vi "niSYS - SA - UTIL - IQ Waveform to TDMS.vi"(8 "error in (no error)":errorcluster, 9 "File Path or Name":path, 11 "Complex Waveform":cluster{"x0":dbl, "dx":dbl, "y":cdb[]} {"y" format="%.2f"; "dx" format="%^.2e"; "x0" format="%^.2e"}) -> (0 "error out":errorcluster)   [LabVIEW 2020]
doc: "(c) Copyright 2006, National Instruments, Inc. This VI may not be duplicated, sold, or distributed without written consent from National Instruments."
panel:
  in  "Waveform Name":string="test"
  in  "Headroom, dB (-1 = Auto)":dbl format="%.1f"
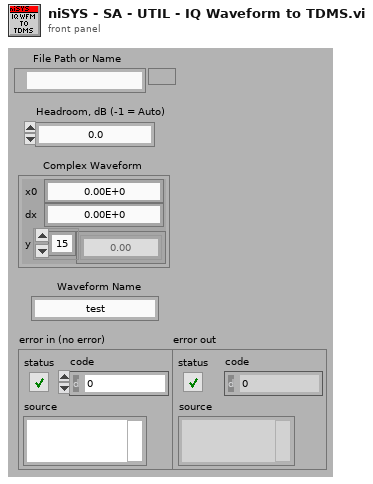
[diagram p1: front panel]
types:
  T1 = enum16{"open", "open or create", "create or replace", "create", "open (read-only)"}
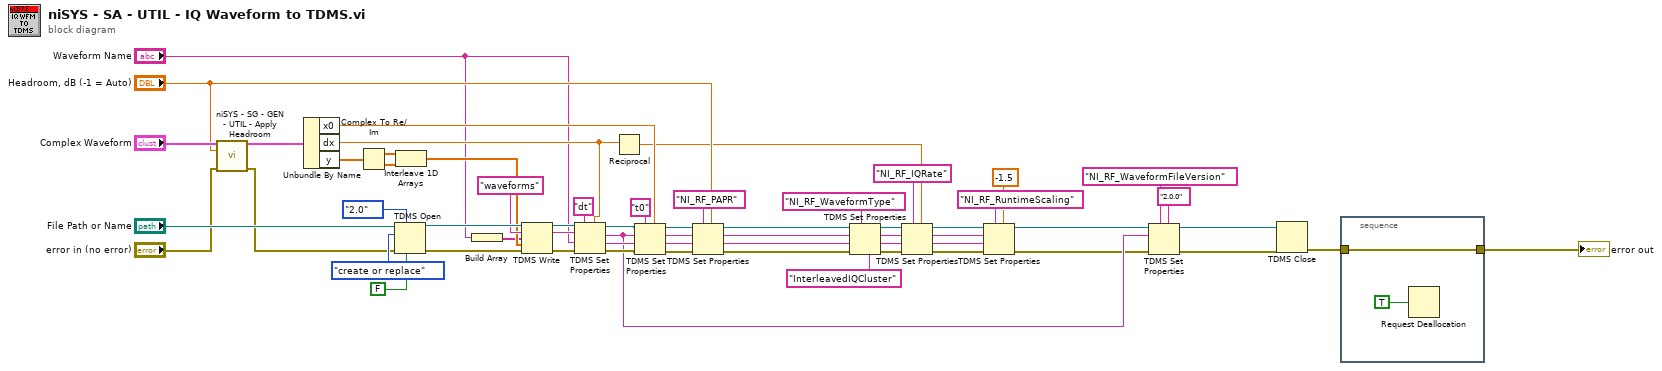
[diagram p0: block diagram]
diagram:
  n1 = call "niSYS - SG - GEN - UTIL - Apply Headroom.vi"("Complex Signal In"="Complex Waveform", "Headroom, dB (-1 = Auto)"="Headroom, dB (-1 = Auto)", "error in (no error)"="error in (no error)") -> ("Complex Signal Out"=w32:cluster{"x0":dbl, "dx":dbl, "y":cdb[]}, "error out"=w29:errorcluster)  [unwired: 10 in, 1 out]
  n2 = Unbundle By Name(w32) -> ("x0"=w36:dbl, "dx"=w27:dbl, "y"=w37:cdb[])
  n3 = Complex To Re/Im(x + iy=w37) -> (x=w39:dbl[], y=w38:dbl[])
  n4 = TDMS Open(6:FALSE ("disable buffering? (T)"), 7:enum16{"1.0", "2.0"}."2.0" ("file format version (2.0)"), 8:w29, 10:T1."create or replace" ("operation (0:open)"), 11:"File Path or Name") -> (0:w51:errorcluster, 3:w52:refnum<k34>)  [unwired: 2 in]
  n5 = Interleave 1D Arrays(w39, w38) -> (w25:dbl[])
  n6 = Build Array("Waveform Name") -> (w19:string[])
  n7 = TDMS Write(0:w52, 5:"waveforms" ("group name"), 7:w19, 9:w25, 11:w51) -> (4:w53:refnum<k34>, 6:w54:string, 15:w28:errorcluster)  [unwired: 1 in, 1 out]
  n8 = TDMS Set Properties(5:w27, 7:"dt", 8:w28, 9:"Waveform Name", 10:w54, 11:w53) -> (0:w49:errorcluster, 1:w44:string, 2:w9:string, 3:w50:refnum<k34>)
  n9 = Reciprocal(x=w27) -> (1/x=w26:dbl)
  n10 = TDMS Set Properties(5:w36, 7:"t0" ("element"), 8:w49, 9:w44, 10:w9, 11:w50) -> (0:w48:errorcluster, 1:w47:string, 2:w46:string, 3:w45:refnum<k34>)
  n11 = TDMS Set Properties(5:"Headroom, dB (-1 = Auto)", 7:"NI_RF_PAPR", 8:w48, 9:w47, 10:w46, 11:w45) -> (0:w14:errorcluster, 1:w15:string, 2:w17:string, 3:w16:refnum<k34>)
  n12 = TDMS Set Properties(5:"InterleavedIQCluster", 7:"NI_RF_WaveformType", 8:w14, 9:w15, 10:w17, 11:w16) -> (0:w24:errorcluster, 1:w3:string, 2:w4:string, 3:w23:refnum<k34>)
  n13 = TDMS Set Properties(5:w26, 7:"NI_RF_IQRate", 8:w24, 9:w3, 10:w4, 11:w23) -> (0:w7:errorcluster, 3:w8:refnum<k34>)  [unwired: 2 out]
  n14 = TDMS Set Properties(5:-1.5, 7:"NI_RF_RuntimeScaling", 8:w7, 9:w3, 10:w4, 11:w8) -> (0:w5:errorcluster, 3:w6:refnum<k34>)  [unwired: 2 out]
  n15 = TDMS Set Properties(5:"2.0.0", 7:"NI_RF_WaveformFileVersion", 8:w5, 10:w9, 11:w6) -> (0:w13:errorcluster, 3:w12:refnum<k34>)  [unwired: 1 in, 2 out]
  n16 = TDMS Close(8:w13, 11:w12) -> (0:w34:errorcluster)  [unwired: 1 out]
  n17 = stacked-sequence {
    tunnel: [w59] -> w58
    tunnel: w34 -> [w59]
    frame #0 {
      n18 = Request Deallocation(TRUE ("flag")) -> ()
    }
  }
  "error out" <- w58
